vi "Teleop.vi"(10 "Match Info":T1={"Autonomous Elapsed Seconds"=0.0, "TeleOp Elapsed Seconds"=0.0, "Disabled Elapsed Seconds"=0.0, "Visited Autonomous"=FALSE, "Visited TeleOp"=FALSE, "Visited Disabled"=FALSE, "Autonomous Settings"={"Autonomous Style"=enum."Independent", "VI Refnum"=refnum}}, 11 "Call Context":T2) -> ()   [LabVIEW 2014]
doc: "This VI is called for each TeleOp packet received from the DS where the robot is not disabled. It is often used to read from the joysticks and update I/O or to update setpoints for timed control loops. It should complete and return within 20 milliseconds or it may miss DS packets."
uses:
  <vilib>/Rock Robotics/WPI/DriverStation/WPI_DriverStationDerivedRobotMode.ctl
  <vilib>/Rock Robotics/WPI/DriverStation/WPI_DriverStationMatch Info.ctl
  Common Code/Solenoid Command.ctl
  Drivetrain Code/Drivetrain Control.ctl
  Drivetrain Code/Drivetrain Mode.ctl
  <vilib>/Rock Robotics/WPI/Joystick/WPI_JoystickGetSetRefNum.vi
  Robot Global Data.vi
  <vilib>/Rock Robotics/Network Tables/SD Write Numeric Array.vi
  <vilib>/Rock Robotics/Network Tables/SD Write Boolean Array.vi
  <vilib>/Rock Robotics/Network Tables/SD Read Number.vi
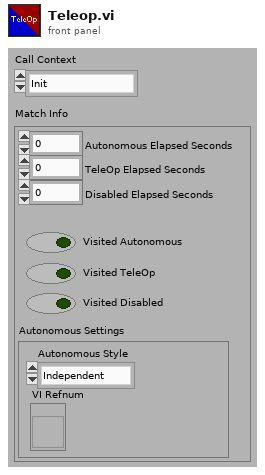
[diagram p1: front panel]
types:
  T1 = typedef "WPI_DriverStationMatch Info.ctl" = cluster{"Autonomous Elapsed Seconds":dbl, "TeleOp Elapsed Seconds":dbl, "Disabled Elapsed Seconds":dbl, "Visited Autonomous":bool, "Visited TeleOp":bool, "Visited Disabled":bool, "Autonomous Settings":cluster{"Autonomous Style":enum16{"Iterative", "Independent"}, "VI Refnum":refnum<vi>}}
  T2 = typedef "WPI_DriverStationDerivedRobotMode.ctl" = enum16{"Init", "Execute", "Stop"}
  T3 = typedef "Drivetrain Control.ctl" = cluster{"Mode":T4, "X":dbl, "Y":dbl, "Heading Target":dbl, "Y Target":dbl}
  T4 = typedef "Drivetrain Mode.ctl" = enum16{"Manual", "Gyro Steer", "Vision Steer", "Drive Distance"}
  T5 = typedef "Solenoid Command.ctl" = cluster{"Lift":bool, "Gripper":bool}
  T6 = typedef "WPI_JoystickDevRef.ctl" = cluster{"Device":T7}
  T7 = typedef "WPI_JoystickDeviceEnum.ctl" = enum16{"USB 0", "USB 1", "USB 2", "USB 3", "USB 4", "USB 5"}
  T8 = cluster{"Buttons[0]":bool, "Buttons[1]":bool, "Buttons[2]":bool, "Buttons[3]":bool, "Buttons[4]":bool, "Buttons[5]":bool, "Buttons[6]":bool, "Buttons[7]":bool, "Buttons[8]":bool}
  T9 = cluster{"Axes[0]":dbl, "Axes[1]":dbl, "Axes[2]":dbl, "Axes[3]":dbl, "Axes[4]":dbl, "Axes[5]":dbl, "Axes[6]":dbl, "Axes[7]":dbl, "Axes[8]":dbl}
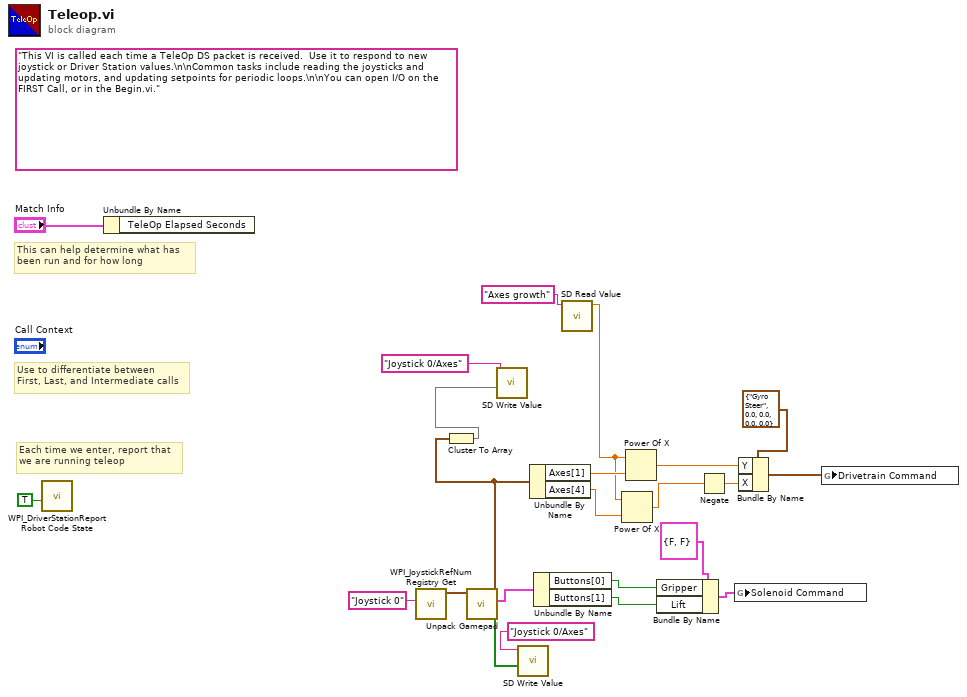
[diagram p0: block diagram]
diagram:
  (unwired) "This VI is called each time a TeleOp DS packet is received.  Use it to respond to new joystick or Driver Station values.\n\nCommon tasks include reading the joysticks and updating motors, and updating setpoints for periodic loops.\n\nYou can open I/O on the FIRST Call, or in the Begin.vi."
  # "Each time we enter, report that\nwe are running teleop"
  # "Use to differentiate between\nFirst, Last, and Intermediate calls"
  # "This can help determine what has\nbeen run and for how long"
  n1 = call <vilib>:"WPI_DriverStationReport Robot Code State.vi"("TeleOp"=TRUE ("Autonomous")) -> ()  [unwired: 10 in, 1 out]
  n2 = Unbundle By Name("Match Info") -> ()  [unwired: 1 out]
  n3 = call <vilib>:"WPI_JoystickRefNum Registry Get.vi"("refnum name"="Joystick 0") -> ("JoystickDevRef"=w20:T6)  [unwired: 9 in, 1 out]
  n4 = call "Unpack Gamepad.vi"("JoystickDevRef"=w20) -> ("Button Array"=w8:bool[], "Button Cluster"=w19:T8, "Axes"=w12:T9)  [unwired: 7 in, 1 out]
  n5 = Cluster To Array(cluster=w12) -> (array=w10:dbl[])
  n6 = call-poly <vilib>:"SD Write Value.vi"("Numeric Array"=w10, "Name"="Joystick 0/Axes") -> ()  [unwired: 8 in, 2 out]
  n7 = call-poly <vilib>:"SD Write Value.vi"("Boolean Array"=w8, "Name"="Joystick 0/Axes") -> ()  [unwired: 8 in, 2 out]
  n8 = Unbundle By Name(w12) -> ("Axes[1]"=w3:dbl, "Axes[4]"=w4:dbl)
  n9 = Unbundle By Name(w19) -> ("Buttons[0]"=w18:bool, "Buttons[1]"=w17:bool)
  n10 = call-poly <vilib>:"SD Read Value.vi"("Name"="Axes growth") -> ("Numeric"=w1:dbl)  [unwired: 8 in, 2 out]
  n11 = Power Of X(1:w4, 2:w1) -> (0:w7:dbl)
  n12 = Power Of X(1:w3, 2:w1) -> (0:w5:dbl)
  n13 = Bundle By Name(cluster=T5 {"Lift"=FALSE, "Gripper"=FALSE} ("Solenoid Command"), "Gripper"=w18, "Lift"=w17) -> (w15:T5)
  n14 = Negate(x=w7) -> (-x=w6:dbl)
  n15 = global write "Robot Global Data.vi" "Solenoid Command"(w15) -> ()
  n16 = Bundle By Name(cluster=T3 {"Mode"=enum."Gyro Steer", "X"=0.0, "Y"=0.0, "Heading Target"=0.0, "Y Target"=0.0} ("Drivetrain Command"), "Y"=w5, "X"=w6) -> (w13:T3)
  n17 = global write "Robot Global Data.vi" "Drivetrain Command"(w13) -> ()
